vi "Iniciar.vi"(0 "VISA resource name":refnum<visa-resource-name>, 1 "baud rate (9600)":u32=9600) -> (2 "Disponible":bool, 3 "VISA resource name 2":refnum<visa-resource-name>, 4 "error out":errorcluster)   [LabVIEW 2015, in "Arduino GIERM.lvlib"]
uses:
  <vilib>/Instr/_visa.llb/VISA Configure Serial Port (Instr).vi
  <instrlib>/Arduino GIERM/Arduino GIERM.lvlib
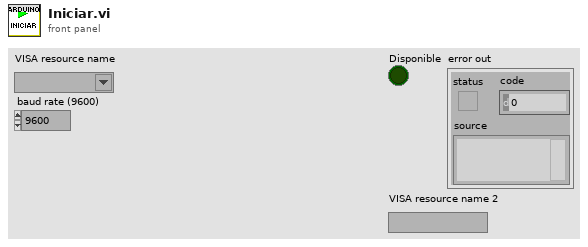
[diagram p1: front panel]
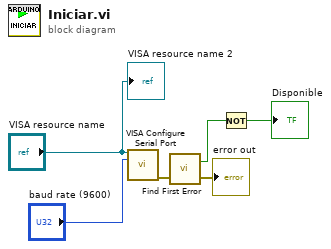
[diagram p0: block diagram]
diagram:
  n1 = call-poly "VISA Configure Serial Port"("VISA resource name"="VISA resource name", "baud rate (9600)"="baud rate (9600)") -> ("error out"=w4:errorcluster)  [unwired: 12 in, 1 out]
  n2 = call <vilib>:"Find First Error.vi"("error in (no error)"=w4) -> ("error out"=→"error out":errorcluster, "error?"=w3:bool)  [unwired: 3 in]
  n3 = Not(x=w3) -> (.not. x?=→"Disponible":bool)
  "VISA resource name 2" <- "VISA resource name"
